vi "tsdb_get_flexray_signal_properties_by_address_verbose.vi"(8 "error in (no error)":errorcluster caption="错误输入（无错误）", 10 "AAddr":string, 11 "path in":path) -> (0 "error out":errorcluster caption="错误输出", 1 "flexray_signal_properties":T1 {"ACompuMethod" items=["fcmIdentical", "fcmLinear", "fcmScaleLinear", "fcmTextTable", "fcmTABNoIntp", "fcmFormula"]; "ASignalType" items=["stCANSignal", "stLINSignal", "stSystemVar", "stFlexRay", "stEthernet"]}, 2 "function return":i32, 3 "path out":path)   [LabVIEW 2014]
doc: "TSAPI(s32)tsdb_get_flexray_signal_properties_by_address_verbose(const char* AAddr,s32* ADBIndex,s32* AECUIndex,s32* AFrameIndex,s32* ASignalIndex,bool* AIsTx,TSignalType* ASignalType,TFlexRayCompuMethod* ACompuMethod,bool* AIsIntel,s32* AActualStartBit,s32* AActualUpdateBit,s32* ALength,double* AFactor,double* AOffset,double* AInitValue,const ppchar AName,const ppchar AComment);"
uses:
  Typedef/FlexRay/flexray_signal_properties.ctl
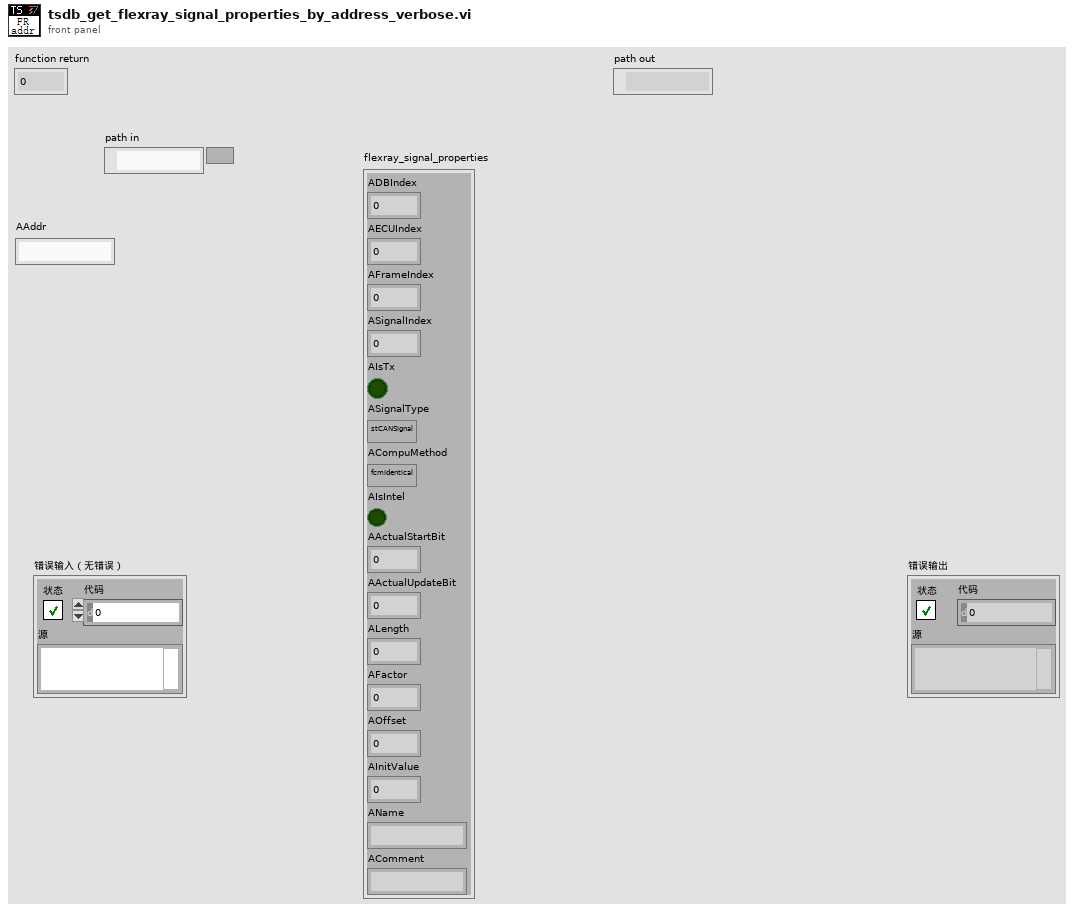
[diagram p1: front panel]
types:
  T1 = typedef "flexray_signal_properties.ctl" = cluster{"ADBIndex":i32, "AECUIndex":i32, "AFrameIndex":i32, "ASignalIndex":i32, "AIsTx":bool, "ASignalType":u32, "ACompuMethod":u32, "AIsIntel":bool, "AActualStartBit":i32, "AActualUpdateBit":i32, "ALength":i32, "AFactor":dbl, "AOffset":dbl, "AInitValue":dbl, "AName":string, "AComment":string}
  T2 = cluster{"ADBIndex":i32, "AECUIndex":i32, "AFrameIndex":i32, "ASignalIndex":i32, "AIsTx":bool, "ASignalType":u32, "ACompuMethod":u32, "AIsIntel":bool, "AActualStartBit":i32, "AActualUpdateBit":i32, "ALength":i32, "AFactor":dbl, "AOffset":dbl, "AInitValue":dbl, "AName":string, "AComment":string}
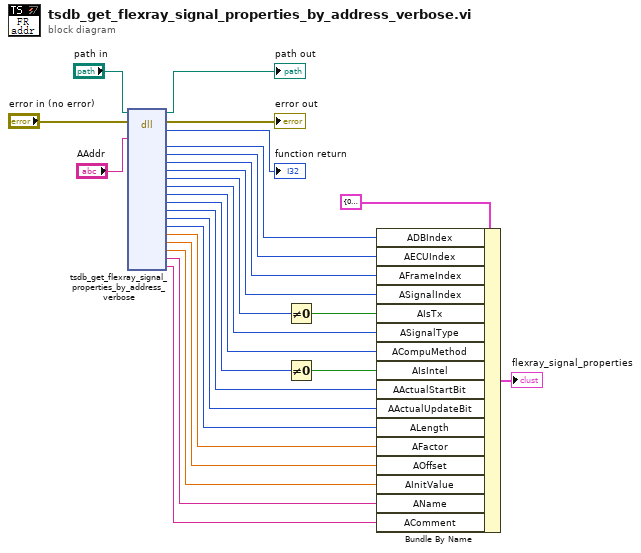
[diagram p0: block diagram]
diagram:
  n1 = dll-call lib="D:/Work/LabVIEW Code/TSMaster Labview SDK/LabVIEW/LabVIEW-TSMasterAPI_CLN/TSMasterAPI_LabVIEW-2024-10-08 14-20-13/Not_organized_vi/TSMaster.*" fn="tsdb_get_flexray_signal_properties_by_address_verbose"(path in="path in", error in="error in (no error)", "AAddr"="AAddr") -> (path out=→"path out":path, error out=→"error out":errorcluster, "返回类型"=→"function return":i32, "ADBIndex"=w16:i32, "AECUIndex"=w15:i32, "AFrameIndex"=w14:i32, "ASignalIndex"=w13:i32, "AIsTx"=w24:u8, "ASignalType"=w11:u32, "ACompuMethod"=w10:u32, "AIsIntel"=w23:u8, "AActualStartBit"=w8:i32, "AActualUpdateBit"=w7:i32, "ALength"=w6:i32, "AFactor"=w5:dbl, "AOffset"=w4:dbl, "AInitValue"=w3:dbl, "AName"=w2:string, "AComment"=w1:string)  [unwired: 18 in]
  n2 = Not Equal To 0?(x=w24) -> (x != 0?=w12:bool)
  n3 = Not Equal To 0?(x=w23) -> (x != 0?=w9:bool)
  n4 = Bundle By Name(cluster=T2 {"ADBIndex"=0, "AECUIndex"=0, "AFrameIndex"=0, "ASignalIndex"=0, "AIsTx"=FALSE, "ASignalType"=0, "ACompuMethod"=0, "AIsIntel"=FALSE, "AActualStartBit"=0, "AActualUpdateBit"=0, "ALength"=0, "AFactor"=0.0, "AOffset"=0.0, "AInitValue"=0.0, "AName"="", "AComment"=""} ("flexray_signal_properties"), "ADBIndex"=w16, "AECUIndex"=w15, "AFrameIndex"=w14, "ASignalIndex"=w13, "AIsTx"=w12, "ASignalType"=w11, "ACompuMethod"=w10, "AIsIntel"=w9, "AActualStartBit"=w8, "AActualUpdateBit"=w7, "ALength"=w6, "AFactor"=w5, "AOffset"=w4, "AInitValue"=w3, "AName"=w2, "AComment"=w1) -> (→"flexray_signal_properties":T2)
